vi "NI-Embedded CAN for RIO subVI - CAN Frame to Table1.vi"(7 "Hexadecimal?":bool, 8 "error in (no error)":errorcluster, 9 "timestamp":timestamp, 10 "CAN frame":T1 {"type" items=["CAN Data", "CAN Remote"]; "identifier" format="%.0x"}, 11 "Old CAN Frames":string[][](array[string])) -> (3 "New CAN Frames":string[][](array[string]), 4 "Iloœæ wiadomoœci CAN odebranych":dbl)   [LabVIEW 2015]
doc: "This example shows how to put a CAN transceiver to sleep on RIO Embedded CAN devices."
uses:
  <vilib>/RioEmbeddedCAN/RioEmbeddedCAN.llb/CANFrameControl.ctl
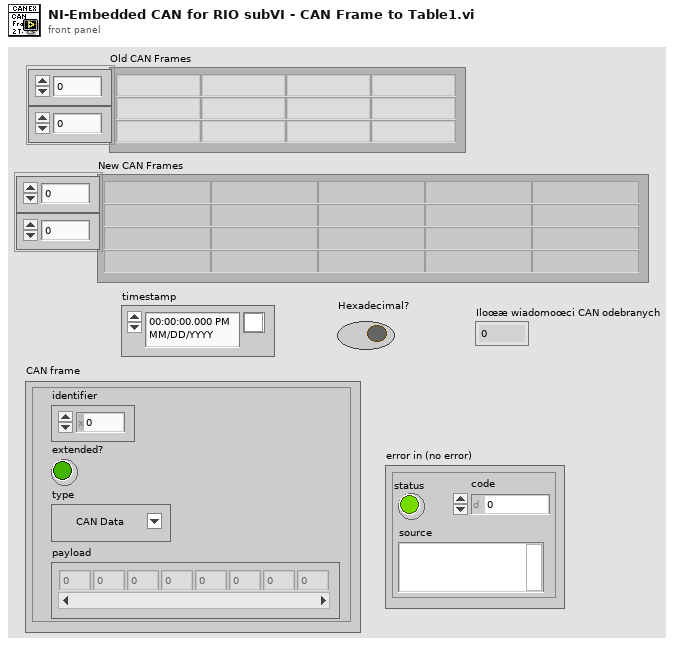
[diagram p1: front panel]
types:
  T1 = typedef "CANFrameControl.ctl" = cluster{"identifier":u32, "extended?":bool, "type":u8, "payload":u8[]}
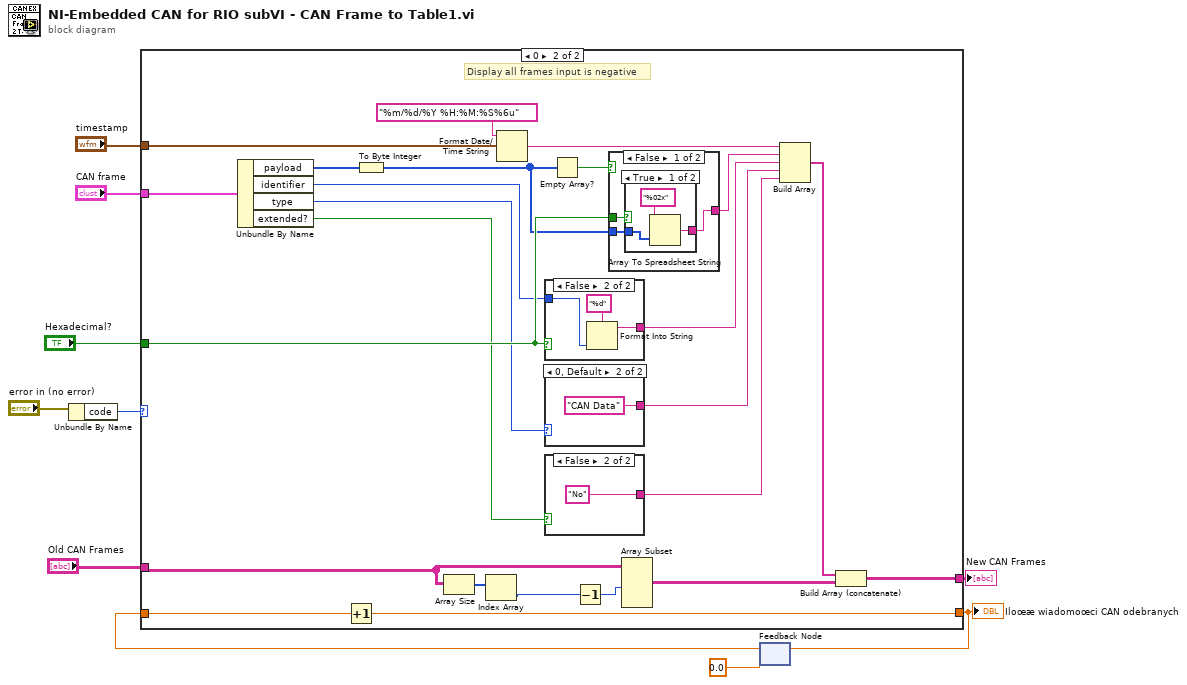
[diagram p0: block diagram]
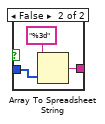
[diagram p3: hidden frame]
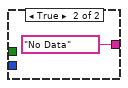
[diagram p4: hidden frame]
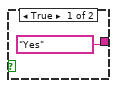
[diagram p5: hidden frame]
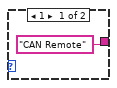
[diagram p6: hidden frame]
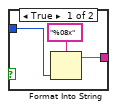
[diagram p7: hidden frame]
diagram:
  n1 = Unbundle By Name("error in (no error)") -> ("code"=w1:i32)
  n2 = feedback #1(0.0) -> (w4:dbl)
  n3 = case shown="0" w1 {
    tunnel: "Old CAN Frames" -> [w12 w35]
    tunnel: [w12 w13] -> w6
    tunnel: "Hexadecimal?" -> [_ w34]
    tunnel: "CAN frame" -> [_ w31]
    tunnel: "timestamp" -> [_ w16]
    tunnel: [w11 w33] -> w5
    tunnel: w4 -> [w11 w32]
    frame Default {
    }
    frame 0 {
      # "Display all frames input is negative"
      n4 = Unbundle By Name(w31) -> ("payload"=w14:u8[], "identifier"=w17:u32, "type"=w24:u8, "extended?"=w21:bool)
      n5 = Increment(x=w32) -> (x+1=w33:dbl)
      n6 = To Byte Integer(number=w14) -> (8bit integer=w15:i8[])
      n7 = Array Size(array=w35) -> (size(s)=w36:i32[])
      n8 = Index Array(array=w36) -> (element=w29:i32)  [unwired: 1 in]
      n9 = Format Date/Time String(time format string (%c)="%m/%d/%Y %H:%M:%S%6u", seconds (now)=w16) -> (date/time string=w26:string)  [unwired: 1 in]
      n10 = case shown="False" w34 {
        tunnel: w17 -> [w52 w56]
        tunnel: [w51 w55] -> w25
        frame True {
          n11 = Format Into String(format string="%08x", w52) -> (resulting string=w51:string)  [unwired: 2 in, 1 out]
        }
        frame False {
          n12 = Format Into String(format string="%d", w56) -> (resulting string=w55:string)  [unwired: 2 in, 1 out]
        }
      }
      n13 = case shown="0, Default" w24 {
        tunnel: ["CAN Remote" "CAN Data"] -> w23
        frame 1 {
        }
        frame 0, Default {
        }
      }
      n14 = case shown="False" w21 {
        tunnel: ["Yes" "No"] -> w22
        frame True {
        }
        frame False {
        }
      }
      n15 = Empty Array?(array=w15) -> (empty?=w18:bool)
      n16 = Decrement(x=w29) -> (x-1=w30:i32)
      n17 = case shown="False" w18 {
        tunnel: [w37 "No Data"] -> w20
        tunnel: w15 -> [w39 _]
        tunnel: w34 -> [w38 _]
        frame False {
          n18 = case shown="True" w38 {
            tunnel: w39 -> [w40 w43]
            tunnel: [w41 w44] -> w37
            frame True {
              n19 = Array To Spreadsheet String(array=w40, 3:"%02x" ("format string")) -> (spreadsheet string=w41:string)  [unwired: 1 in]
            }
            frame False {
              n20 = Array To Spreadsheet String(array=w43, 3:"%3d" ("format string")) -> (spreadsheet string=w44:string)  [unwired: 1 in]
            }
          }
        }
        frame True {
        }
      }
      n21 = Array Subset(array=w35, length (row)=w30) -> (w27:string[][])  [unwired: 3 in]
      n22 = Build Array(w26, w20, w25, w23, w22) -> (w28:string[])
      n23 = Build Array (concatenate)(w28, w27) -> (w13:string[][])
    }
  }
  "New CAN Frames" <- w6
  "Iloœæ wiadomoœci CAN odebranych" <- w5
  n24 = feedback-in #1(w5) -> ()
